vi "cRIO_ZNB_AMI_INICIALIZAR.vi"(8 "error in (no error)":errorcluster, 11 "User event":T1) -> (0 "error out":errorcluster)   [LabVIEW 2017]
uses:
  DISPLAY/UserEventReference.ctl
  DISPLAY/UserEventData.ctl
  DISPLAY/DataType.ctl
  DISPLAY/Display_Command Control.ctl
panel:
  out "STATUS":string
  # "Input"
  # "Output"
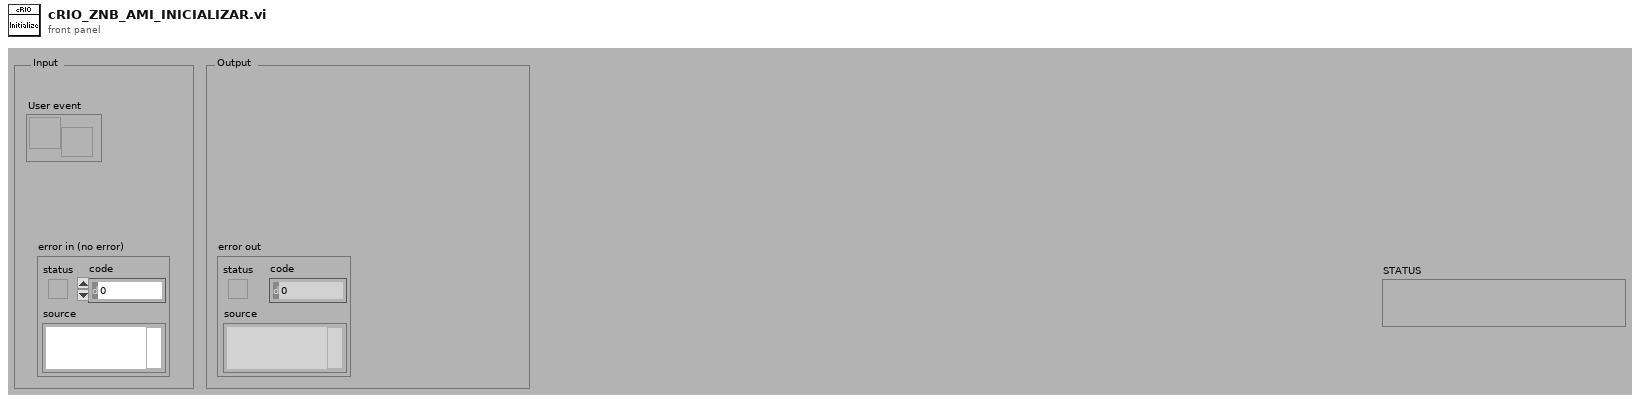
[diagram p1: front panel]
types:
  T1 = typedef "UserEventReference.ctl" = refnum<user-event>
  T2 = typedef "DataType.ctl" = enum16{"Initialize Front Panel", "Update Front Panel", "Update Graph", "Enable/Disable Controls", "Update Status"}
  T3 = typedef "Display_Command Control.ctl" = enum16{"Initialize", "Generate Event", "Shutdown"}
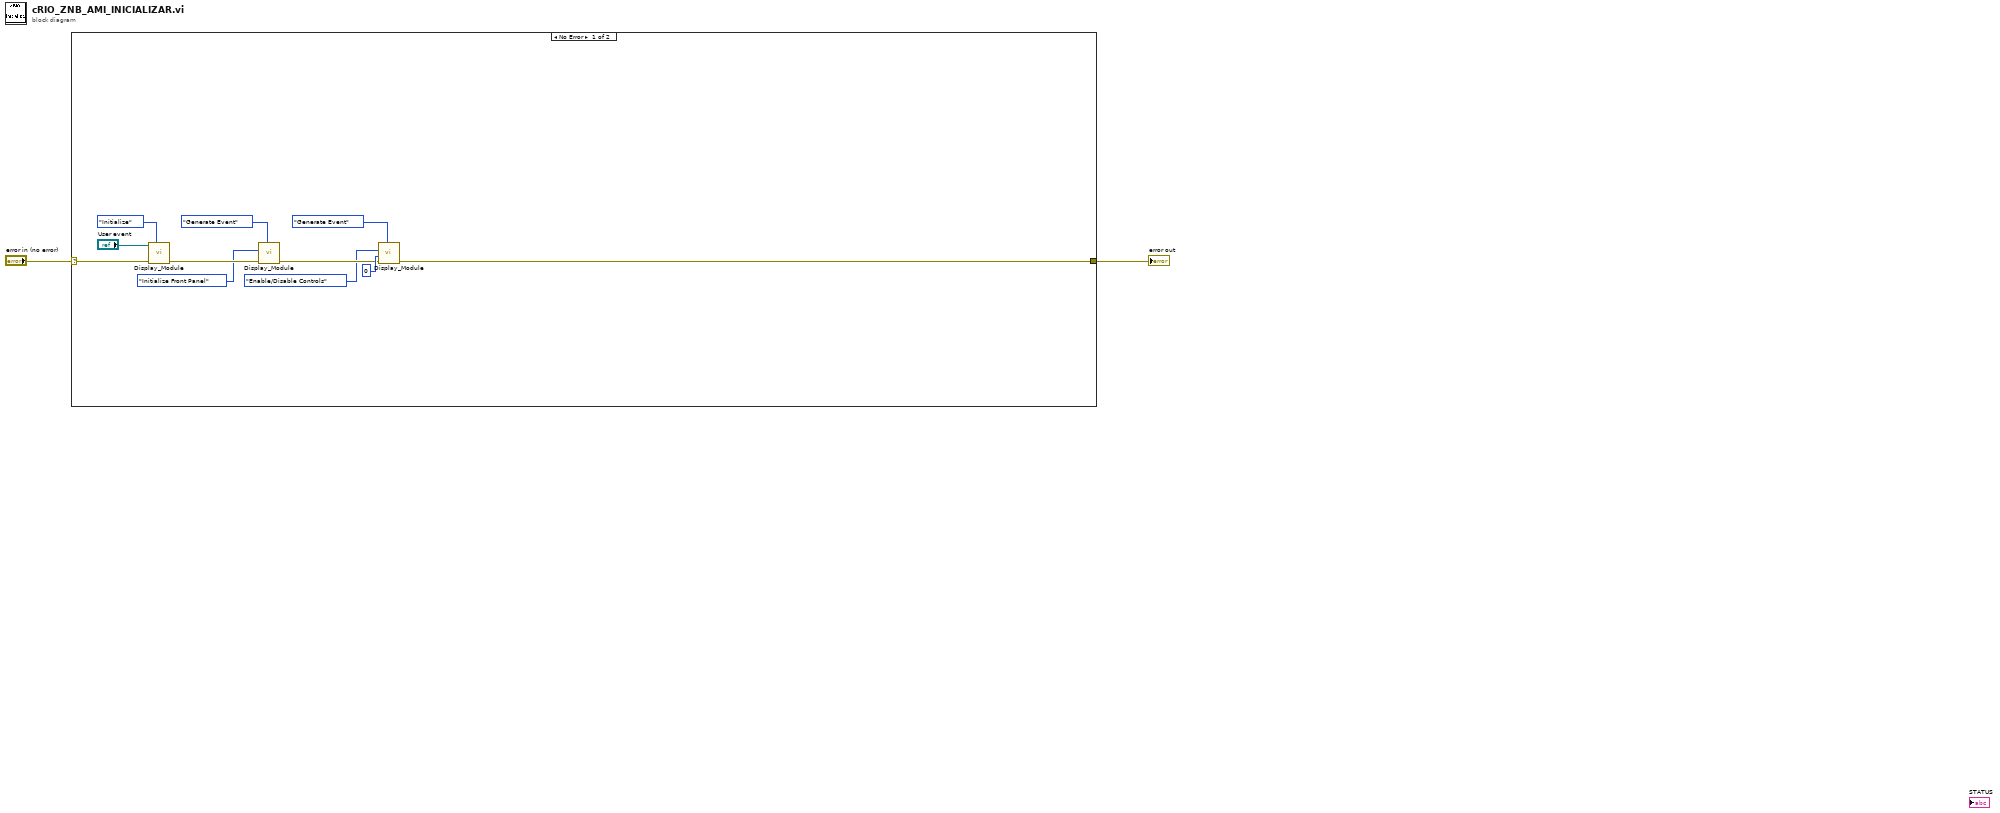
[diagram p0: block diagram]
diagram:
  n1 = case shown="No Error" "error in (no error)" {
    selector: "error in (no error)" -> [w4 w14]
    tunnel: [w3 w14] -> w1
    frame No Error {
      n2 = call "Display_Module.vi"("Command"=Display_Command_Control."Initialize", "error in (no error)"=w4, "user event out"="User event") -> ("error out"=w11:errorcluster)  [unwired: 8 in]
      n3 = call "Display_Module.vi"("Command"=Display_Command_Control."Generate Event", "error in (no error)"=w11, "Data Type"=DataType."Initialize Front Panel") -> ("error out"=w10:errorcluster)  [unwired: 8 in]
      n4 = call "Display_Module.vi"("Command"=Display_Command_Control."Generate Event", "error in (no error)"=w10, "Data"=0, "Data Type"=DataType."Enable/Disable Controls") -> ("error out"=w3:errorcluster)  [unwired: 7 in]
    }
    frame Error {
    }
  }
  "error out" <- w1
